vi "非空数组的时间戳写入 (子VI).vi"(0 "CODMn":string, 1 "氨氮":string, 2 "电导率":string, 3 "水温":string, 4 "浊度":string, 5 "DO":string, 6 "叶绿素":string, 7 "PH":string, 8 "总氮":string, 9 "总磷":string, 11 "藻密度":string, 17 "CODCr":string) -> (20 "字符串 5":string)   [LabVIEW 2016]
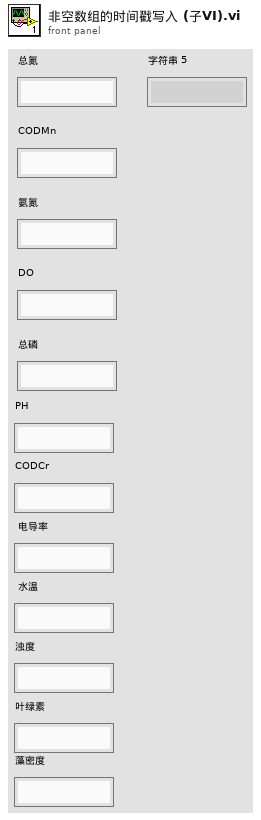
[diagram p1: front panel]
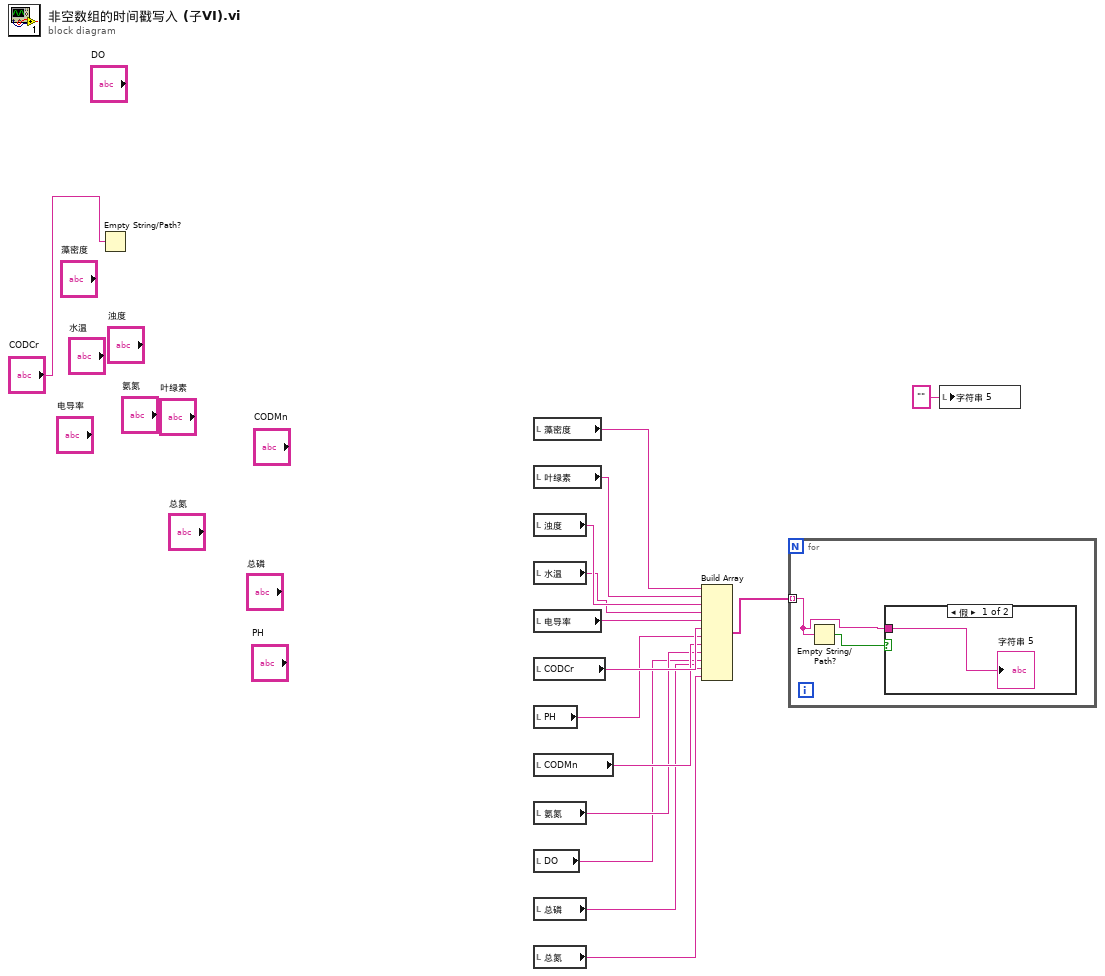
[diagram p0: block diagram]
diagram:
  n1 = Empty String/Path?(string/path="CODCr") -> ()  [unwired: 1 out]
  n2 = local read "藻密度"() -> (w14:string)
  n3 = local read "叶绿素"() -> (w13:string)
  n4 = local read "浊度"() -> (w12:string)
  n5 = local read "水温"() -> (w11:string)
  n6 = local read "电导率"() -> (w10:string)
  n7 = local read "CODCr"() -> (w9:string)
  n8 = local read "PH"() -> (w8:string)
  n9 = local read "CODMn"() -> (w7:string)
  n10 = local read "氨氮"() -> (w6:string)
  n11 = local read "DO"() -> (w5:string)
  n12 = local read "总磷"() -> (w4:string)
  n13 = local read "总氮"() -> (w3:string)
  n14 = Build Array(w14, w13, w12, w11, w10, w9, w8, w7, w6, w5, w4, w3) -> (w2:string[])
  n15 = for {
    tunnel: w2 -> [w16] mode=indexing
    n16 = Empty String/Path?(string/path=w16) -> (empty?=w17:bool)
    n17 = case shown="假" w17 {
      tunnel: w16 -> [w18 _]
      frame False {
        "字符串 5" <- w18
      }
      frame True {
      }
    }
  }
  n18 = local write "字符串 5"("" ("字符串 5")) -> ()
